vi "testUintSquare.vi"(8 "error in (no error)":errorcluster, 11 "TestCase in":refnum<class "UnitTestUintClass.lvclass">) -> (0 "error out":errorcluster, 3 "TestCase out":refnum<class "UnitTestUintClass.lvclass">)   [LabVIEW 2011, in "UnitTestUintClass.lvclass"]
uses:
  UnitTestUintClass.lvclass
  UnitTestUintClass.lvclass/UnitTestUintClass.ctl
  <vilib>/addons/_JKI Toolkits/VI Tester/TestCase.llb/TestCase.lvclass
  UintClass/UintClass.lvclass
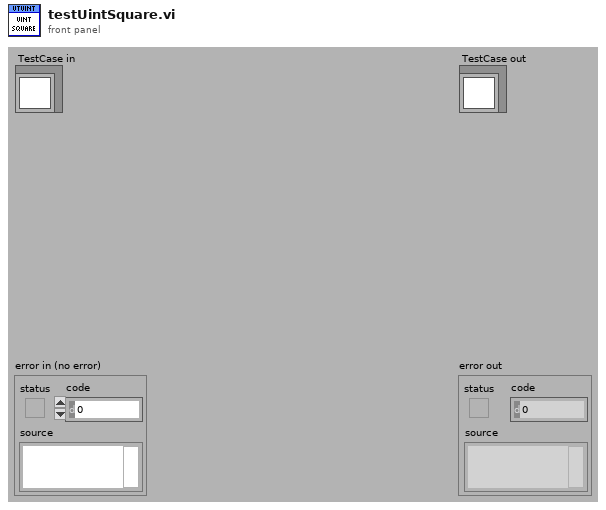
[diagram p1: front panel]
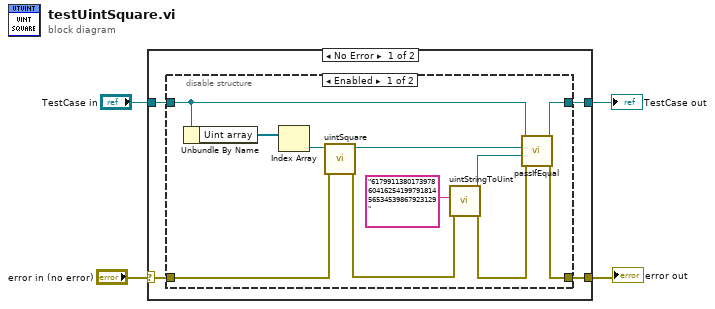
[diagram p0: block diagram]
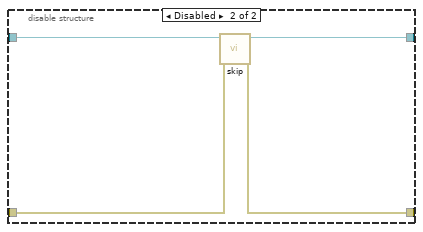
[diagram p2: hidden frame]
diagram:
  n1 = case shown="No Error" "error in (no error)" {
    selector: "error in (no error)" -> [w6 w25]
    tunnel: [w5 w25] -> w3
    tunnel: [w7 w24] -> w1
    tunnel: "TestCase in" -> [w8 w24]
    frame No Error {
      n2 = disable-structure shown="Enabled" {
        disable-tunnel: w8 -> [w17 w23]
        disable-tunnel: [w19 w20] -> w7
        disable-tunnel: w6 -> [w11 w22]
        disable-tunnel: [w18 w21] -> w5
        frame Enabled {
          n3 = Unbundle By Name(w17) -> ("Uint array"=w16:refnum<class "UintClass.lvclass">[])
          n4 = Index Array(array=w16) -> (element=w15:refnum<class "UintClass.lvclass">)  [unwired: 1 in]
          n5 = call "uintSquare.vi"("Error in (no error)"=w11, "Int in"=w15) -> ("Error out"=w12:errorcluster, "pow(Int, 2)"=w14:refnum<class "UintClass.lvclass">)  [unwired: 7 in, 1 out]
          n6 = call "uintStringToUint.vi"("Error in (no error)"=w12, "String in"="61799113801739786041625419979181456534539867923129") -> ("Error out"=w10:errorcluster, "Uint out"=w13:refnum<class "UintClass.lvclass">)  [unwired: 8 in]
          n7 = call-dynamic "passIfEqual.vi"("error in (no error)"=w10, "y"=w13, "x"=w14, "TestCase in"=w17) -> ("error out"=w18:errorcluster, "TestCase out"=w19:refnum<class "UnitTestUintClass.lvclass">)  [unwired: 6 in]
        }
        frame Disabled {
          n8 = call <vilib>:"skip.vi"("error in (no error)"=w22, "TestCase in"=w23) -> ("error out"=w21:errorcluster, "TestCase out"=w20:refnum<class "UnitTestUintClass.lvclass">)  [unwired: 8 in]
        }
      }
    }
    frame Error {
    }
  }
  "error out" <- w3
  "TestCase out" <- w1
